vi "UA_XML_OP.vi"(8 "error in (no error)":errorcluster caption="error in", 10 "xml Raw Data":string[](array[string])) -> (0 "error out":errorcluster, 1 "XML Data Out":T2[][](array[typedef]), 3 "Server config info":T1)   [LabVIEW 2013, in "CreateOPCUAServerAuto.lvlib"]
uses:
  CreateOPCUAServerAuto.lvlib
  UA_XML Data.ctl
  UA_RowType.ctl
  UA_Server config info.ctl
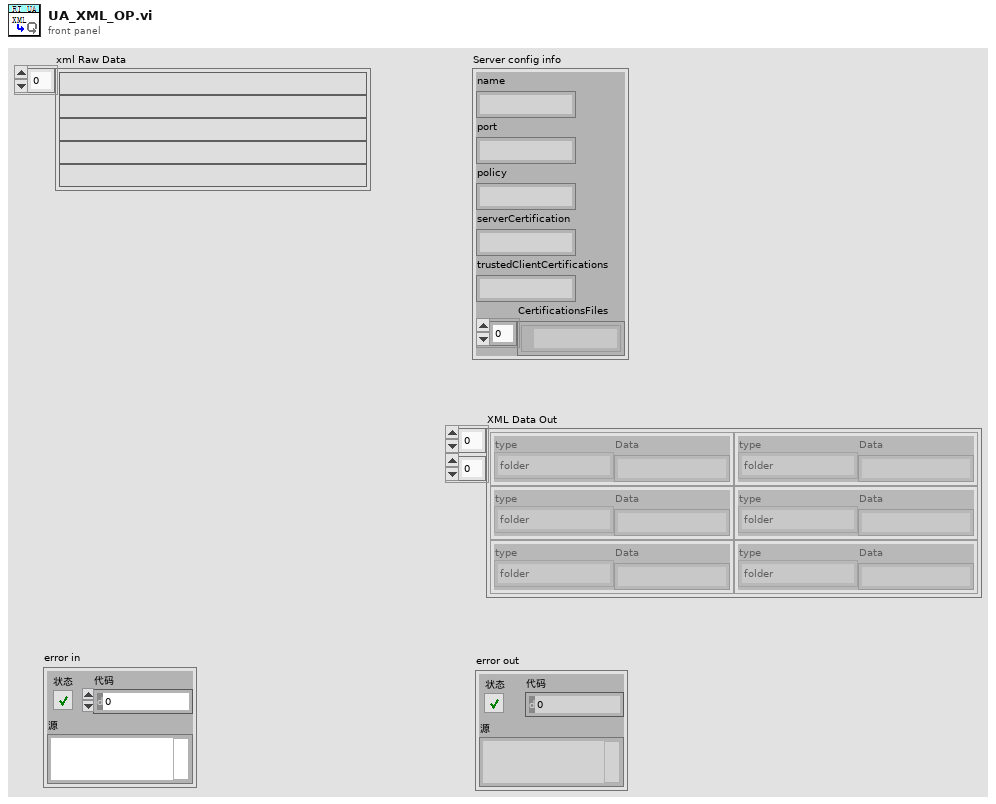
[diagram p1: front panel]
types:
  T1 = typedef "CreateOPCUAServerAuto.lvlib/UA_Server config info.ctl" = cluster{"name":string, "port":string, "policy":string, "serverCertification":string, "trustedClientCertifications":string, "CertificationsFiles":path[]}
  T2 = typedef "CreateOPCUAServerAuto.lvlib/UA_XML Data.ctl" = cluster{"type":T3, "Data":string}
  T3 = typedef "CreateOPCUAServerAuto.lvlib/UA_RowType.ctl" = enum16{"none", "folder", "item", "property", "folder end", "item end"}
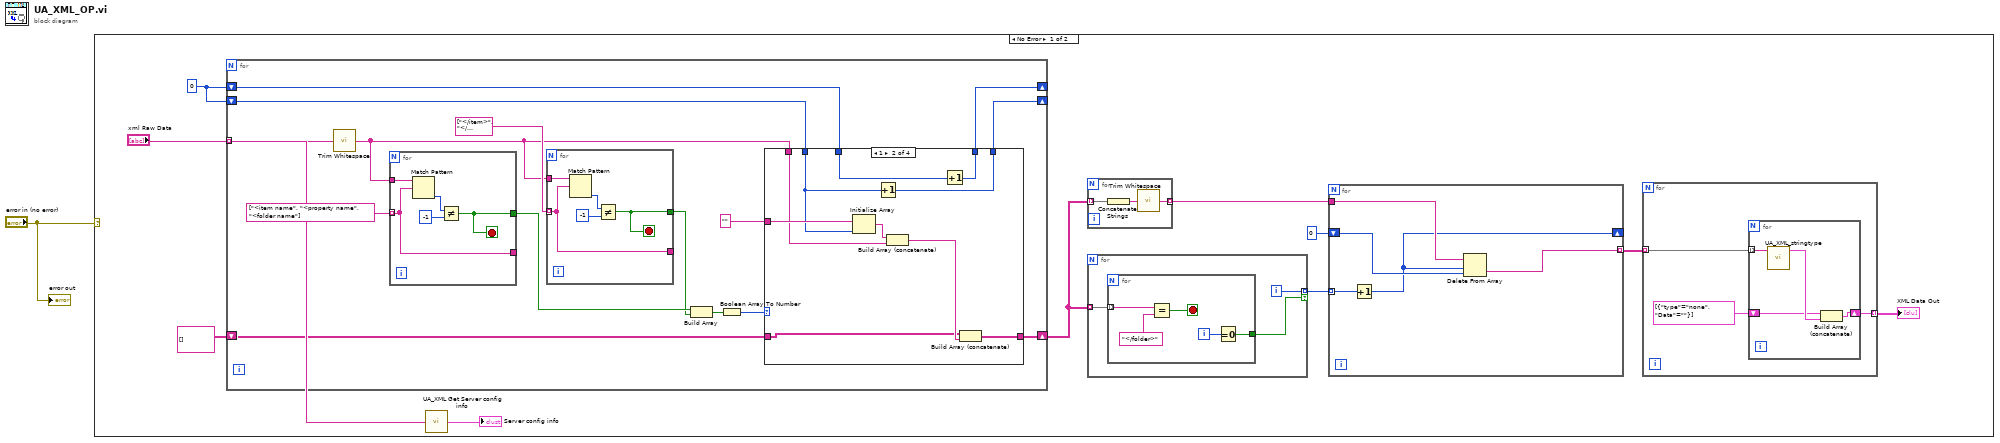
[diagram p0: block diagram]
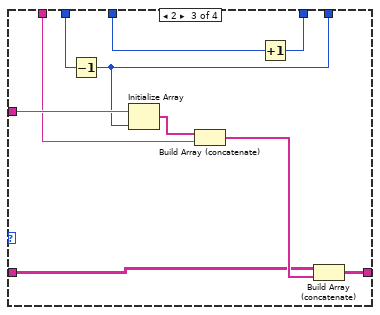
[diagram p3: hidden frame]
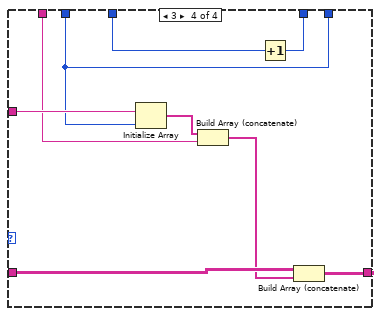
[diagram p4: hidden frame]
diagram:
  n1 = case shown="No Error" "error in (no error)" {
    frame No Error {
      w5 = 0
      n2 = for {
        tunnel: "xml Raw Data" -> [w16] mode=indexing
        shift-right: [w24] -> _
        shift-left: w5 -> [w21]
        shift-right: [w23] -> _
        shift-left: w5 -> [w20]
        shift-right: [w12] -> w6
        shift-left: string[][] [] -> [w13]
        n3 = call <vilib>:"Trim Whitespace.vi"("string"=w16) -> ("trimmed string"=w15:string)  [unwired: 1 in]
        n4 = for {
          tunnel: w15 -> [w68]
          tunnel: string[] ["<item name", "<property name", "<folder name"] ("start string") -> [w64] mode=indexing
          tunnel: [w65] -> w19
          tunnel: [w64] -> _
          stop <- w65 stop-if-true
          n5 = Match Pattern(string=w68, regular expression=w64) -> (offset past match=w67:i32)  [unwired: 1 in, 3 out]
          n6 = Not Equal?(x=w67, y=-1) -> (x != y?=w65:bool)
        }
        n7 = for {
          tunnel: w15 -> [w63]
          tunnel: string[] ["</item>", "</property>", "</folder>"] ("end string") -> [w59] mode=indexing
          tunnel: [w60] -> w18
          tunnel: [w59] -> _
          stop <- w60 stop-if-true
          n8 = Match Pattern(string=w63, regular expression=w59) -> (offset past match=w62:i32)  [unwired: 1 in, 3 out]
          n9 = Not Equal?(x=w62, y=-1) -> (x != y?=w60:bool)
        }
        n10 = Build Array(w19, w18) -> (w17:bool[])
        n11 = Boolean Array To Number(Boolean array=w17) -> (number=w22:u32)
        n12 = case shown="1" w22 {
          tunnel: [w29 w39 w49 w58] -> w24
          tunnel: [w28 w38 w45 w55] -> w23
          tunnel: w21 -> [w29 w36 w47 w57]
          tunnel: w20 -> [w28 w30 w48 w55]
          tunnel: w15 -> [_ w34 w43 w53]
          tunnel: "" -> [_ w37 w46 w56]
          tunnel: w13 -> [w27 w31 w41 w52]
          tunnel: [w27 w32 w40 w50] -> w12
          frame 0, Default {
          }
          frame 1 {
            n13 = Initialize Array(w37, w30) -> (w35:string[])
            n14 = Increment(x=w30) -> (x+1=w38:i32)
            n15 = Build Array (concatenate)(w35, w34) -> (w33:string[])
            n16 = Increment(x=w36) -> (x+1=w39:i32)
            n17 = Build Array (concatenate)(w31, w33) -> (w32:string[][])
          }
          frame 2 {
            n18 = Decrement(x=w48) -> (x-1=w45:i32)
            n19 = Initialize Array(w46, w45) -> (w44:string[])
            n20 = Build Array (concatenate)(w44, w43) -> (w42:string[])
            n21 = Increment(x=w47) -> (x+1=w49:i32)
            n22 = Build Array (concatenate)(w41, w42) -> (w40:string[][])
          }
          frame 3 {
            n23 = Initialize Array(w56, w55) -> (w54:string[])
            n24 = Build Array (concatenate)(w54, w53) -> (w51:string[])
            n25 = Increment(x=w57) -> (x+1=w58:i32)
            n26 = Build Array (concatenate)(w52, w51) -> (w50:string[][])
          }
        }
      }
      n27 = call "UA_XML Get Server config info.vi"("xml Raw Data"="xml Raw Data") -> ("Server config info"=→"Server config info":T1)
      n28 = for {
        tunnel: w6 -> [w71] mode=indexing
        tunnel: [w70] -> w11 mode=indexing if=w69
        i -> [w70]
        n29 = for {
          tunnel: w71 -> [w76] mode=indexing
          tunnel: [w72] -> w69
          i -> [w73]
          stop <- w74 stop-if-true
          n30 = Equal?(x=w76, y="</folder>") -> (x = y?=w74:bool)
          n31 = Equal To 0?(x=w73) -> (x = 0?=w72:bool)
        }
      }
      n32 = for {
        tunnel: [w91] -> w10 mode=indexing
        tunnel: w6 -> [w90] mode=indexing
        n33 = Concatenate Strings(w90) -> (w89:string)
        n34 = call <vilib>:"Trim Whitespace.vi"("string"=w89) -> ("trimmed string"=w91:string)  [unwired: 1 in]
      }
      n35 = for {
        tunnel: w11 -> [w86] mode=indexing
        tunnel: w10 -> [w88]
        shift-right: [w84] -> _
        shift-left: 0 -> [w87]
        tunnel: [w85] -> w8 mode=indexing
        n36 = Increment(x=w86) -> (x+1=w84:i32)
        n37 = Delete From Array(array=w88, length=w84, index=w87) -> (deleted portion=w85:string[])  [unwired: 1 out]
      }
      n38 = for {
        tunnel: w8 -> [w79] mode=indexing
        tunnel: [w77] -> w7 mode=indexing
        n39 = for {
          tunnel: w79 -> [w83] mode=indexing
          shift-right: [w80] -> w77
          shift-left: T2[] [{"type"=enum."none", "Data"=""}] -> [w81]
          n40 = call "UA_XML_stringtype.vi"("XML String"=w83) -> ("XML Data"=w82:T2[])  [unwired: 10 in]
          n41 = Build Array (concatenate)(w81, w82) -> (w80:T2[])
        }
      }
      "XML Data Out" <- w7
    }
    frame Error {
    }
  }
  "error out" <- "error in (no error)"
